vi "StraightDrivePID.vi"(6 "PID Constants":T1={"proportional gain (Kc)"=0.015, "integral time (Ti, min)"=0.001, "derivative time (Td, min)"=0.0} {"derivative time (Td, min)" format="%.3f"; "integral time (Ti, min)" format="%.3f"; "proportional gain (Kc)" format="%.3f"}, 7 "output range":cluster{"output high":dbl, "output low":dbl}={"output high"=1.0, "output low"=-1.0} {"output low" min=-1.0 max=1.0 step=0.1 format="%.2f"; "output high" min=-1.0 max=1.0 step=0.1 format="%.2f"}, 8 "StraightDriveEngage?":bool, 9 "sDriveRate":dbl, 10 "Average Controller Value":dbl, 11 "Controller Value":dbl) -> (3 "Motor Value":dbl)   [LabVIEW 2012]
uses:
  StraightDrivePIDEnum.ctl
  Robot Global Data.vi
  <vilib>/addons/control/pid/pid.llb/PID (DBL).vi
  <vilib>/addons/control/pid/NI_PID_pid.lvlib
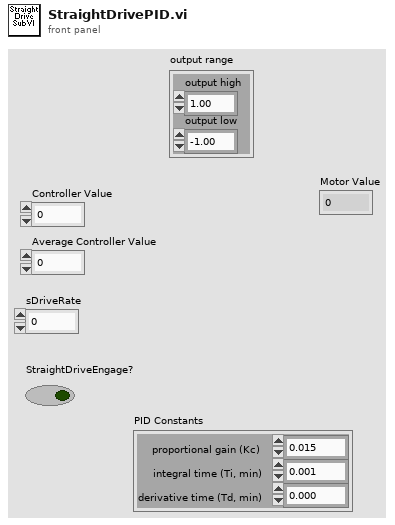
[diagram p1: front panel]
types:
  T1 = cluster{"proportional gain (Kc)":dbl, "integral time (Ti, min)":dbl, "derivative time (Td, min)":dbl}
  T2 = typedef "StraightDrivePIDEnum.ctl" = enum16{"Inactive", "Active"}
  T3 = typedef "LoopDisable.ctl" = cluster{"Climb.vi":bool, "LauncherAngle.vi":bool, "Launcher.vi":bool, "ArmControl.vi":bool, "WinchMotor.vi":bool, "ReadDriveEncoder.vi":bool}
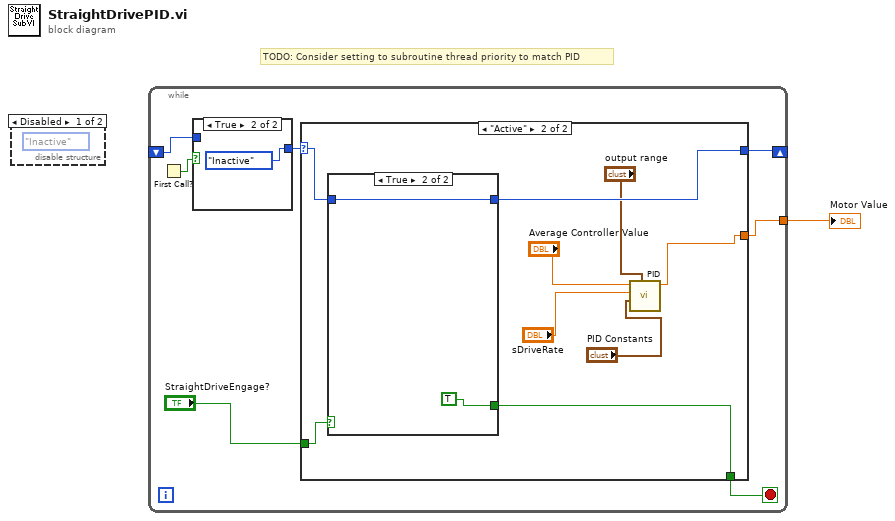
[diagram p0: block diagram]
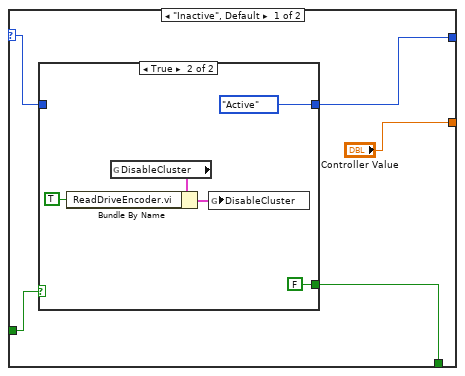
[diagram p4: hidden frame]
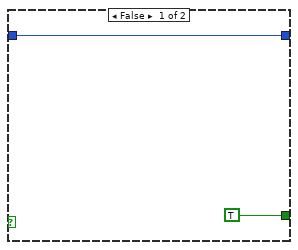
[diagram p5: hidden frame]
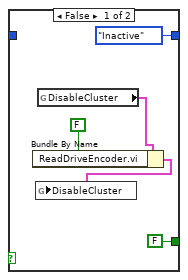
[diagram p6: hidden frame]
diagram:
  # "TODO: Consider setting to subroutine thread priority to match PID"
  n1 = disable-structure shown="Disabled" {
    frame Disabled {
      (unwired) StraightDrivePIDEnum."Inactive"
    }
    frame Enabled {
    }
  }
  n2 = while {
    shift-right: [w7] -> _
    shift-left: _ -> [w3]
    tunnel: [w6] -> w1
    stop <- w8 stop-if-true
    n3 = First Call?() -> (First Call?: T/F=w4:bool)
    n4 = case shown="True" w4 {
      tunnel: [w9 StraightDrivePIDEnum."Inactive"] -> w5
      tunnel: w3 -> [w9 _]
      frame False {
      }
      frame True {
      }
    }
    n5 = case shown="\"Active\"" w5 {
      selector: w5 -> [w14 w30]
      tunnel: [w12 w28] -> w8
      tunnel: "StraightDriveEngage?" -> [w15 w31]
      tunnel: [w13 w29] -> w7
      tunnel: ["Controller Value" w23] -> w6
      frame "Inactive", Default {
        n6 = case shown="True" w15 {
          tunnel: w14 -> [w17 _]
          tunnel: [w17 StraightDrivePIDEnum."Active"] -> w13
          tunnel: [TRUE FALSE] -> w12
          frame False {
          }
          frame True {
            n7 = global read "Robot Global Data.vi" "DisableCluster"() -> (w19:T3)
            n8 = Bundle By Name(cluster=w19, "ReadDriveEncoder.vi"=TRUE) -> (w21:T3)
            n9 = global write "Robot Global Data.vi" "DisableCluster"(w21) -> ()
          }
        }
      }
      frame "Active" {
        n10 = case shown="True" w31 {
          tunnel: w30 -> [_ w38]
          tunnel: [StraightDrivePIDEnum."Inactive" w38] -> w29
          tunnel: [FALSE TRUE] -> w28
          frame False {
            n11 = global read "Robot Global Data.vi" "DisableCluster"() -> (w33:T3)
            n12 = Bundle By Name(cluster=w33, "ReadDriveEncoder.vi"=FALSE) -> (w35:T3)
            n13 = global write "Robot Global Data.vi" "DisableCluster"(w35) -> ()
          }
          frame True {
          }
        }
        n14 = call-poly <vilib>:"PID.vi"("output range"="output range", "PID gains"="PID Constants", "process variable"="sDriveRate", "setpoint"="Average Controller Value") -> ("output"=w23:dbl)  [unwired: 6 in, 1 out]
      }
    }
  }
  "Motor Value" <- w1
